vi "Add Label.vi"(6 "transfer type":T2, 8 "error in":errorcluster, 9 "SDI value":T3=-1 items=["All"=-1, "0 (b00)"=0, "1 (b01)"=1, "2 (b10)"=2, "3 (b11)"=3], 10 "label value":u32, 11 "port ref":T1 format="%.0x") -> (0 "error out":errorcluster, 2 "label ref":T1 format="%.0x", 3 "port ref out":T1 format="%.0x")   [LabVIEW 2020, in "Ballard ARINC 429 Scripting.lvlib"]
uses:
  Ballard ARINC 429 Scripting.lvlib
  Shared/SDI.ctl
  Shared/Transfer Type.ctl
  <vilib>/NI VeriStand/Custom Device API/Custom Device Item Ref.ctl
  Shared/Label Properties.ctl
  Shared/Label.ctl
  <vilib>/NI VeriStand/Custom Device API/Custom Device Channel.ctl
  <vilib>/NI VeriStand/Custom Device API/Custom Device Channel Type.ctl
  Constants.vi
  <vilib>/NI VeriStand/Custom Device API/Custom Device API.lvlib
  ARINC 429/ARINC 429 Scripting.lvlib
  Import/ARINC 429 Import.lvlib
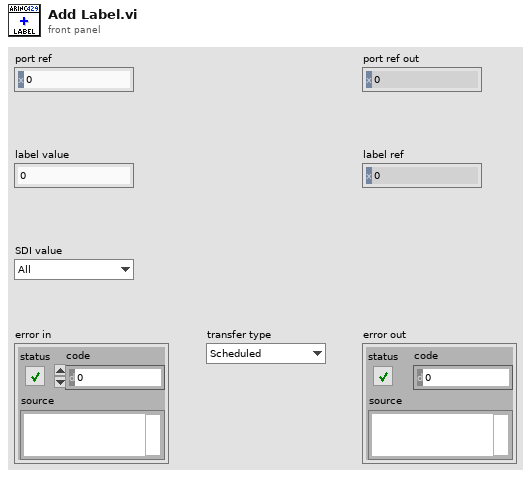
[diagram p1: front panel]
types:
  T1 = typedef "Custom Device API.lvlib/Custom Device Item Ref.ctl" = u64
  T2 = typedef "Transfer Type.ctl" = enum16{"Scheduled", "Acyclic", "Block", "Strobe"}
  T3 = typedef "SDI.ctl" = i32
  T4 = typedef "Label Properties.ctl" = cluster{"label (Dec)":T5, "SDI value":u8, "SDI enabled":bool}
  T5 = typedef "Label.ctl" = u8
  T6 = typedef "Direction.ctl" = enum16{"Rx", "Tx"}
  T7 = typedef "Custom Device API.lvlib/Custom Device Channel.ctl" = cluster{"Type":T8, "Units":string, "Default Value":dbl, "Faultable":bool, "Scalable":bool}
  T8 = typedef "Custom Device API.lvlib/Custom Device Channel Type.ctl" = enum16{"Input", "Output"}
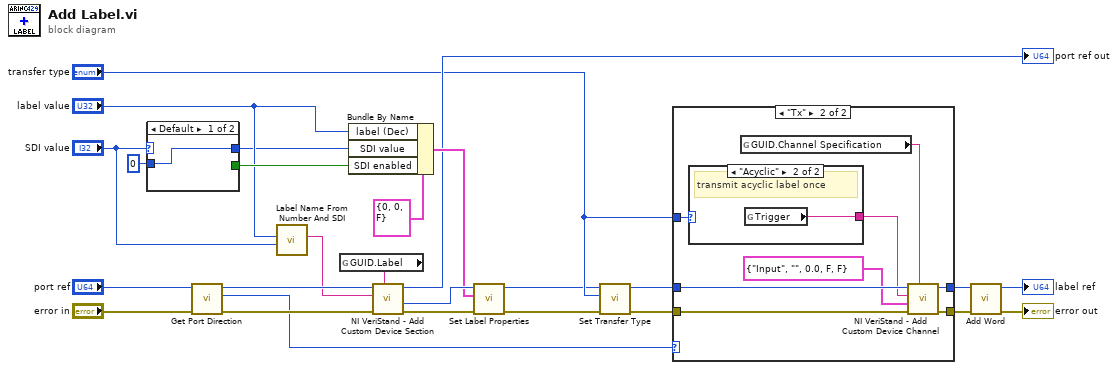
[diagram p0: block diagram]
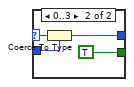
[diagram p2: hidden frame]
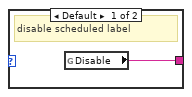
[diagram p4: hidden frame]
diagram:
  n1 = case shown="Default" "SDI value" {
    selector: "SDI value" -> [_ w31]
    tunnel: [w27 w28] -> w2
    tunnel: u8 0 ("SDI value") -> [w27 w30]
    tunnel: [_ TRUE] -> w9
    frame Default {
    }
    frame 0..3 {
      n2 = Coerce To Type(0:w31, 1:w30) -> (2:w28:u8)
    }
  }
  n3 = call "Get Port Direction.vi"("error in"="error in", "port ref in"="port ref") -> ("error out"=w12:errorcluster, "direction"=w11:T6, "port ref out"=w13:T1)  [unwired: 7 in]
  n4 = call "Label Name From Number And SDI.vi"("SDI value"="SDI value", "label (Dec)"="label value") -> ("label name"=w4:string)  [unwired: 9 in]
  n5 = global read "Constants.vi" "GUID.Label"() -> (w19:string)
  n6 = Bundle By Name(cluster=T4 {"label (Dec)"=0, "SDI value"=0, "SDI enabled"=FALSE} ("label properties"), "label (Dec)"="label value", "SDI value"=w2, "SDI enabled"=w9) -> (w16:T4)
  n7 = call <vilib>:"NI VeriStand - Add Custom Device Section.vi"("GUID (Default Section)"=w19, "error in (no error)"=w12, "Section Name"=w4, "Parent Ref in"=w13) -> ("error out"=w21:errorcluster, "Section Ptr"=w20:T1, "Parent Ref out"=→"port ref out":T1)  [unwired: 4 in, 1 out]
  n8 = call "Set Label Properties.vi"("error in"=w21, "label properties"=w16, "label ref"=w20) -> ("error out"=w22:errorcluster, "label ref out"=w5:T1)  [unwired: 7 in]
  n9 = call "Set Transfer Type.vi"("error in"=w22, "transfer type"="transfer type", "label ref in"=w5) -> ("error out"=w23:errorcluster, "label ref out"=w25:T1)  [unwired: 7 in]
  n10 = case shown="\"Tx\"" w11 {
    tunnel: w23 -> [w32 w41]
    tunnel: [w32 w40] -> w24
    tunnel: w25 -> [w33 w39]
    tunnel: [w33 w38] -> w26
    tunnel: "transfer type" -> [_ w36]
    frame "Rx", Default {
    }
    frame "Tx" {
      n11 = case shown="\"Acyclic\"" w36 {
        tunnel: [w42 w43] -> w35
        frame Default {
          # "disable scheduled label"
          n12 = global read "Constants.vi" "Disable"() -> (w42:string)
        }
        frame "Acyclic" {
          # "transmit acyclic label once"
          n13 = global read "Constants.vi" "Trigger"() -> (w43:string)
        }
      }
      n14 = global read "Constants.vi" "GUID.Channel Specification"() -> (w37:string)
      n15 = call <vilib>:"NI VeriStand - Add Custom Device Channel.vi"("GUID (Default Channel)"=w37, "error in (no error)"=w41, "Channel"=T7 {"Type"=enum."Input", "Units"="", "Default Value"=0.0, "Faultable"=FALSE, "Scalable"=FALSE}, "Channel Name"=w35, "Parent Ref in"=w39) -> ("error out"=w40:errorcluster, "Parent Ref out"=w38:T1)  [unwired: 3 in, 2 out]
    }
  }
  n16 = call "Add Word.vi"("error in"=w24, "label ref"=w26) -> ("error out"=→"error out":errorcluster, "label ref out"=→"label ref":T1)  [unwired: 6 in, 2 out]
